vi "R4Master.vi"(6 "LabVIEW Web Service":refnum<class "Web Service.lvclass">=refnum) -> ()   [LabVIEW 2016]
uses:
  <vilib>/wsapi/Web Service.lvclass
  R4Controls/R4SBR_SetParams.ctl
  Controls/pH_SetParams Standard.ctl
  <vilib>/Platform/TimedLoop/XDataNode/timing_clust.ctl
  <vilib>/Platform/TimedLoop/XDataNode/nitl_modes.ctl
  <vilib>/Platform/TimedLoop/XDataNode/wakeup.ctl
  <vilib>/Platform/TimedLoop/XDataNode/loadnilvce.vi
  <vilib>/Platform/TimedLoop/XDataNode/XDataNode.xnode
  <vilib>/Platform/TimedLoop/XDataNode/XDNodeRunTimeDep.lvlib
panel:
  out "?":cluster{"Value":dbl, "Value":dbl}(graph)
  in  "R4SBR_Manual":T1
  out "error out":errorcluster
  out "error out (DATA COLLECT)":errorcluster
  out "error out (SBR)":errorcluster
  in  "R4SBR_SetParams":T2=[{"Phase"="Plug Feed", "Time, min"=0.0, "SBR_Manual (Standard)"={"Media Pump"=TRUE, "Water Pump"=TRUE, "Gas Pump"=FALSE, "Effluent Pump"=FALSE, "Release Pump"=FALSE}}, {"Phase"="Mixed Feed", "Time, min"=135.0, "SBR_Manual (Standard)"={"Media Pump"=TRUE, "Water Pump"=TRUE, "Gas Pump"=TRUE, "Effluent Pump"=FALSE, "Release Pump"=FALSE}}, {"Phase"="Mixed w/o Feed", "Time, min"=92.0, "SBR_Manual (Standard)"={"Media Pump"=FALSE, "Water Pump"=FALSE, "Gas Pump"=TRUE, "Effluent Pump"=FALSE, "Release Pump"=FALSE}}, {"Phase"="Settle", "Time, min"=7.0, "SBR_Manual (Standard)"={"Media Pump"=FALSE, "Water Pump"=FALSE, "Gas Pump"=FALSE, "Effluent Pump"=FALSE, "Release Pump"=TRUE}}, {"Phase"="Decant", "Time, min"=5.0, "SBR_Manual (Standard)"={"Media Pump"=FALSE, "Water Pump"=FALSE, "Gas Pump"=FALSE, "Effluent Pump"=TRUE, "Release Pump"=TRUE}}, {"Phase"="Idle", "Time, min"=1.0, "SBR_Manual (Standard)"={"Media Pump"=FALSE, "Water Pump"=FALSE, "Gas Pump"=FALSE, "Effluent Pump"=FALSE, "Release Pump"=FALSE}}]
  in  "R4 SBR_Switch":bool
  in  "R4DOSetParams":T3={"Set Point, mg/L"=0.0, "Tolerance, mg/L"=0.05, "N2 Valve Gain"=5000.0, "Air Valve Gain"=1000.0}
  in  "R4DOManual":cluster{"Air MFC":dbl, "N2 MFC":dbl} {"Air MFC" scale=0.0..500.0; "N2 MFC" scale=0.0..500.0}
  in  "R4 DO_Switch":bool=TRUE
  out "R4DO":cluster{"Signal":dbl, "Value":dbl}={"Signal"=0.012310571769960223, "Value"=5.584491888741017}
  in  "R4 pH_Switch":bool=TRUE
  in  "R4 pH_SetParams":T4={"Set Point"=7.5, "Tolerance"=0.1, "Pump Time On, secs"=6.0}
  in  "R4pH_Manual":cluster{"Acid Pump":bool, "Base Pump":bool}
  out "pH":cluster{"Signal":dbl, "Value":dbl}={"Signal"=0.0127343038254794, "Value"=7.4567616069444576}
  out "Timestamp":string="09/22/2017 10:45:23.660"
  out "Status":string="Off"
  out "Cycle Time Elapsed":dbl
  out "Phase Time Elapsed":dbl
  # "Use the web service input terminal to call the VIs on the Service subpalette of the Web Services palette. Do not remove it from the connector pane unless you don't need access to the palette."
  # "Any additional terminals added to the connector pane of a startup VI will be ignored."
  # "DO Control"
  # "SBR Control"
  # "If On, Automate SBR Cycle"
  # "pH Control"
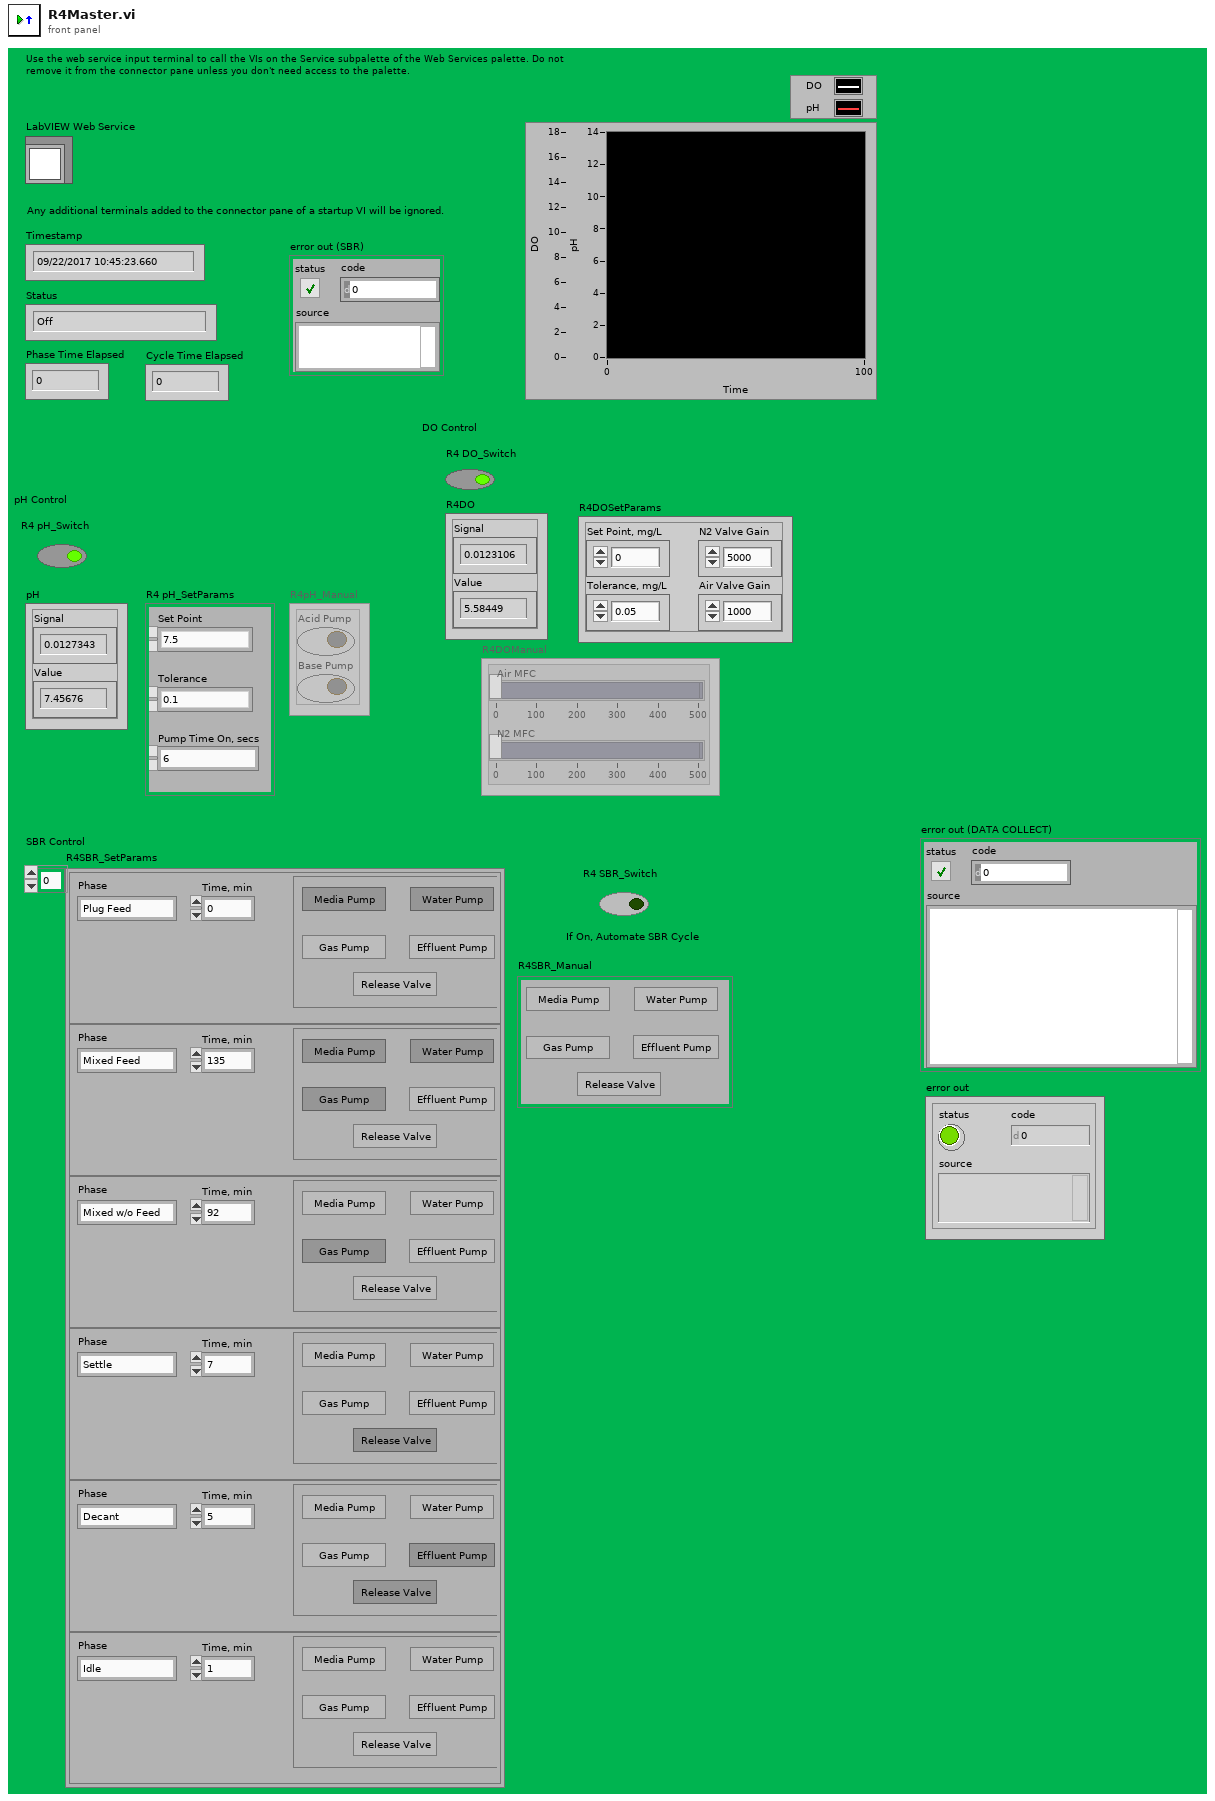
[diagram p1: front panel]
types:
  T1 = cluster{"Media Pump":bool, "Water Pump":bool, "Gas Pump":bool, "Effluent Pump":bool, "Release Pump":bool}
  T2 = typedef "R4SBR_SetParams.ctl" = cluster{"Phase":string, "Time, min":dbl, "SBR_Manual (Standard)":cluster{"Media Pump":bool, "Water Pump":bool, "Gas Pump":bool, "Effluent Pump":bool, "Release Pump":bool}}[]
  T3 = cluster{"Set Point, mg/L":dbl, "Tolerance, mg/L":dbl, "N2 Valve Gain":dbl, "Air Valve Gain":dbl}
  T4 = typedef "pH_SetParams Standard.ctl" = cluster{"Set Point":dbl, "Tolerance":dbl, "Pump Time On, secs":dbl}
  T5 = typedef "XDNodeRunTimeDep.lvlib/timing_clust.ctl" = cluster{"Expected End [f-1]":u64, "Actual End [f-1]":u64, "Finished Late? [f-1]":bool, "Expected End [i-1]":u64, "Actual End [i-1]":u64, "Finished Late? [i-1]":bool, "Expected Start [i]":u64, "Actual Start [i]":u64, "Expected Start [f]":u64, "Actual Start [f]":u64, "Source Name":string, "Structure Name":string, "Period":i64, "Deadline":i64, "Offset":i64, "Start":i64, "Priority":i32, "Timeout":i32, "Mode":T6, "Wakeup Reason":T7, "Error":errorcluster, "Source Type":string, "Secondary Source Type":string, "Global End Time":u64, "Global Start Time":u64, "Frame Duration":u64, "Iteration Duration":u64, "Assigned CPU":i32, "I/O Scan Engine Mode":u32}
  T6 = typedef "XDNodeRunTimeDep.lvlib/nitl_modes.ctl" = enum32{"No Change", "Process missed periods, maintain original phase", "Discard missed periods, maintain original phase", "Process missed periods, ignore original phase", "Discard missed periods, ignore original phase"}
  T7 = typedef "XDNodeRunTimeDep.lvlib/wakeup.ctl" = enum32{"Normal", "Aborted", "Asynchronous wakeup", "Timing source error", "Timed loop error", "Timeout"}
  T8 = cluster{"Media Pump":bool, "Water Pump":bool, "Effluent Pump":bool, "Release Valve":bool, "Gas Pump":bool}
  T9 = enum8{"Enabled", "Disabled", "Disabled and Grayed Out"}
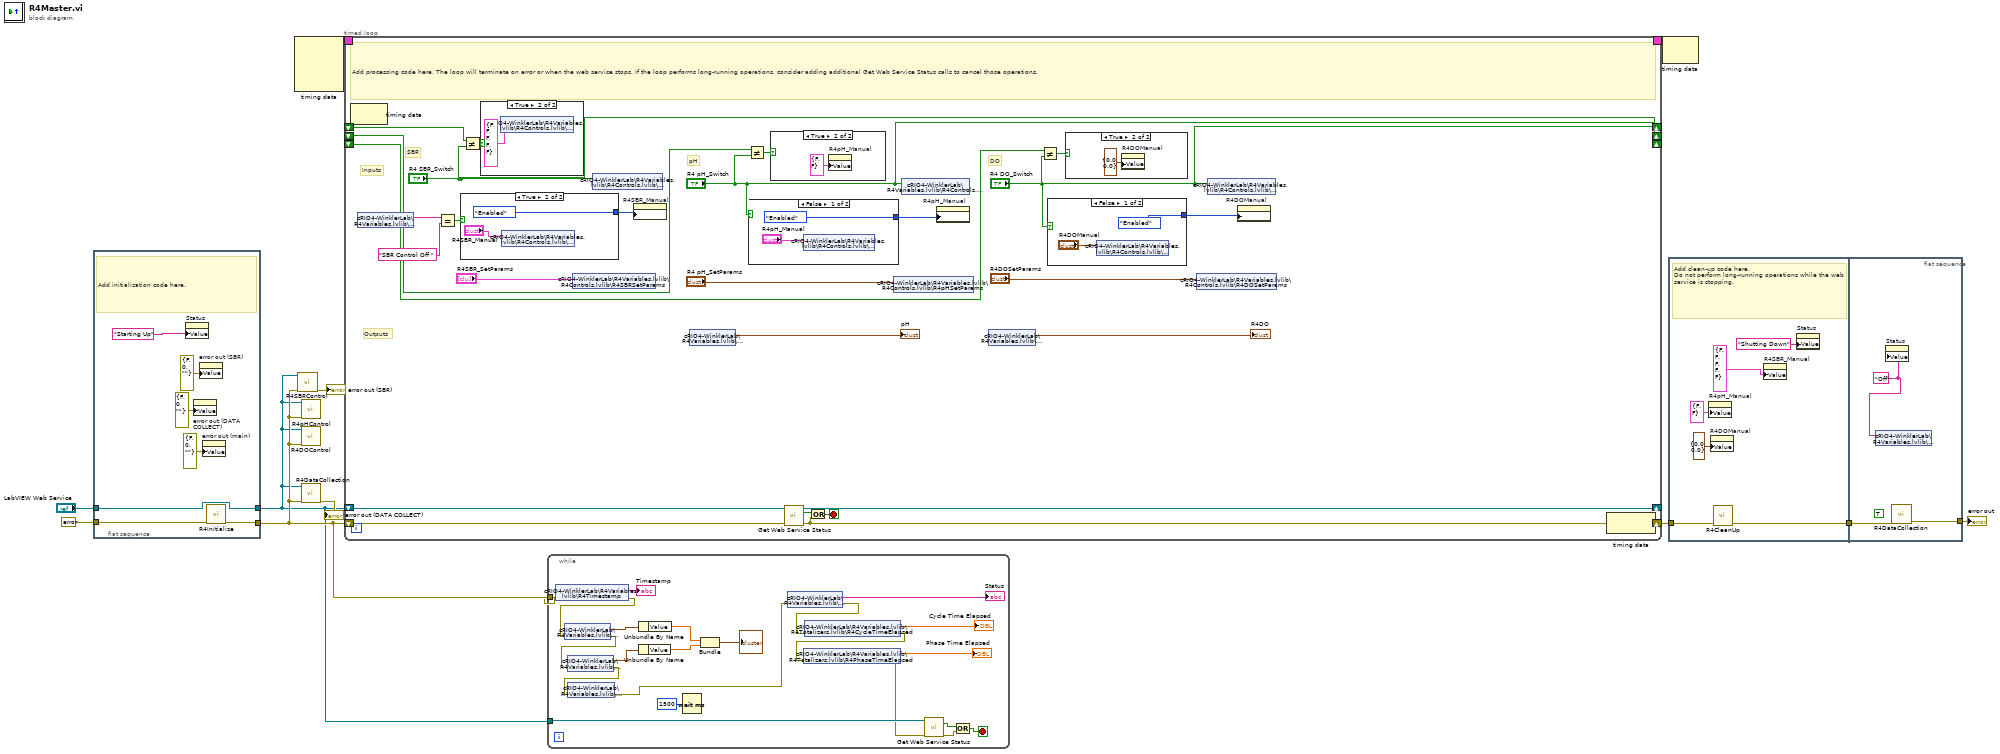
[diagram p0: block diagram]
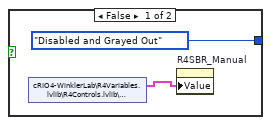
[diagram p5: hidden frame]
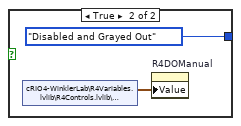
[diagram p6: hidden frame]
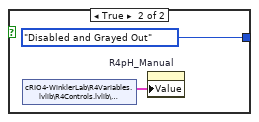
[diagram p7: hidden frame]
diagram:
  n1 = flat-sequence {
    tunnel: "LabVIEW Web Service" -> [w16]
    tunnel: errorcluster {"status"=FALSE, "code"=0, "source"=""} ("error constant") -> [w18]
    tunnel: [w17] -> w3
    tunnel: [w16] -> w1
    frame #0 {
      # "Add initialization code here."
      n2 = property on="Status" class="Str"("Value"="Starting Up" ("Status")) -> ()  [unwired: 2 in, 2 out]
      n3 = property on="error out (DATA COLLECT)" class="Clust (strict)"("Value"=errorcluster {"status"=FALSE, "code"=0, "source"=""} ("error out (DATA COLLECT)")) -> ()  [unwired: 2 in, 2 out]
      n4 = property on="error out (SBR)" class="Clust (strict)"("Value"=errorcluster {"status"=FALSE, "code"=0, "source"=""} ("error out (SBR)")) -> ()  [unwired: 2 in, 2 out]
      n5 = property on="error out (main)" class="Clust (strict)"("Value"=errorcluster {"status"=FALSE, "code"=0, "source"=""} ("error out")) -> ()  [unwired: 2 in, 2 out]
      n6 = call "R4Initialize.vi"("error in (no error)"=w18) -> ("error out"=w17:errorcluster)  [unwired: 10 in]
    }
  }
  n7 = node-c288() -> (w8:T5)  [unwired: 4 in]
  n8 = call "R4SBRControl.vi"("error constant"=w3, "LabVIEW Web Service"=w1) -> ("error out"=→"error out (SBR)":errorcluster)  [unwired: 9 in]
  n9 = call "R4pHControl.vi"("error constant"=w3, "LabVIEW Web Service"=w1) -> ()  [unwired: 10 in]
  n10 = call "R4DOControl.vi"("error constant"=w3, "LabVIEW Web Service"=w1) -> ()  [unwired: 10 in]
  n11 = call "R4DataCollection.vi"("error constant"=w3, "LabVIEW Web Service"=w1) -> ("error out"=→"error out (DATA COLLECT)":errorcluster)  [unwired: 9 in]
  n12 = timed-loop {
    shift-right: [w42] -> w9
    shift-left: w3 -> [w41]
    shift-right: [w39] -> _
    shift-left: w1 -> [w39]
    timing: w8 -> [_]
    timing-out: [_] -> w7
    shift-right: ["R4 SBR_Switch"] -> _
    shift-left: _ -> [w29]
    shift-right: ["R4 pH_Switch"] -> _
    shift-left: _ -> [w35]
    shift-right: ["R4 DO_Switch"] -> _
    shift-left: _ -> [w33]
    stop <- w40 stop-if-true
    # "DO"
    # "pH"
    # "Outputs"
    # "Inputs"
    # "SBR"
    # "Add processing code here. The loop will terminate on error or when the web service stops. If the loop performs long-running operations, consider adding additional Get Web Service Status calls to cancel those operations."
    n13 = node-c288() -> ()  [unwired: 1 in, 1 out]
    n14 = shared-variable "cRIO4-WinklerLab\\R4Variables.lvlib\\R4Status"() -> (w28:string)  [unwired: 1 in, 1 out]
    n15 = Equal?(x=w28, y="SBR Control Off " ("string")) -> (x = y?=w30:bool)
    n16 = case shown="True" w30 {
      tunnel: [T9."Disabled and Grayed Out" ("Disabled") T9."Enabled" ("Disabled")] -> w19
      frame False {
        n17 = shared-variable "cRIO4-WinklerLab\\R4Variables.lvlib\\R4Controls.lvlib\\R4SBRManual"() -> (w47:T1)  [unwired: 1 in, 1 out]
        n18 = property on="R4SBR_Manual" class="Clust (strict)"("Value"=w47) -> ()  [unwired: 2 in, 2 out]
      }
      frame True {
        n19 = shared-variable "cRIO4-WinklerLab\\R4Variables.lvlib\\R4Controls.lvlib\\R4SBRManual"("R4SBR_Manual") -> ()  [unwired: 1 in, 1 out]
      }
    }
    n20 = Not Equal?(x=w29, y="R4 SBR_Switch") -> (x != y?=w36:bool)
    n21 = case shown="True" w36 {
      frame False {
      }
      frame True {
        n22 = shared-variable "cRIO4-WinklerLab\\R4Variables.lvlib\\R4Controls.lvlib\\R4SBRManual"(T8 {"Media Pump"=FALSE, "Water Pump"=FALSE, "Effluent Pump"=FALSE, "Release Valve"=FALSE, "Gas Pump"=FALSE} ("R4SBRManual")) -> ()  [unwired: 1 in, 1 out]
      }
    }
    n23 = shared-variable "cRIO4-WinklerLab\\R4Variables.lvlib\\R4Controls.lvlib\\R4SBRSetParams"("R4SBR_SetParams") -> ()  [unwired: 1 in, 1 out]
    n24 = shared-variable "cRIO4-WinklerLab\\R4Variables.lvlib\\R4Controls.lvlib\\R4SBRSwitch"("R4 SBR_Switch") -> ()  [unwired: 1 in, 1 out]
    n25 = property on="R4SBR_Manual" class="Clust (strict)"("DisabledEnum"=w19) -> ()  [unwired: 2 in, 2 out]
    n26 = shared-variable "cRIO4-WinklerLab\\R4Variables.lvlib\\R4Signals.lvlib\\R4pH"() -> (→"pH":cluster{"Signal":dbl, "Value":dbl})  [unwired: 1 in, 1 out]
    n27 = Not Equal?(x=w35, y="R4 pH_Switch") -> (x != y?=w34:bool)
    n28 = case shown="False" "R4 pH_Switch" {
      tunnel: [T9."Enabled" ("Disabled") T9."Disabled and Grayed Out" ("Disabled")] -> w38
      frame False {
        n29 = shared-variable "cRIO4-WinklerLab\\R4Variables.lvlib\\R4Controls.lvlib\\R4pHManual"("R4pH_Manual") -> ()  [unwired: 1 in, 1 out]
      }
      frame True {
        n30 = shared-variable "cRIO4-WinklerLab\\R4Variables.lvlib\\R4Controls.lvlib\\R4pHManual"() -> (w57:cluster{"Acid Pump":bool, "Base Pump":bool})  [unwired: 1 in, 1 out]
        n31 = property on="R4pH_Manual" class="Clust (strict)"("Value"=w57) -> ()  [unwired: 2 in, 2 out]
      }
    }
    n32 = case shown="True" w34 {
      frame False {
      }
      frame True {
        n33 = property on="R4pH_Manual" class="Clust (strict)"("Value"=cluster{"Acid Pump":bool, "Base Pump":bool} {"Acid Pump"=FALSE, "Base Pump"=FALSE} ("R1pH_Manual")) -> ()  [unwired: 2 in, 2 out]
      }
    }
    n34 = call <vilib>:"Get Web Service Status.vi"("LabVIEW Web Service"=w39, "error in (no error)"=w41) -> ("service stopping?"=w43:bool, "error out"=w42:errorcluster)  [unwired: 11 in, 1 out]
    n35 = Or(x=w43, y=w42) -> (x .or. y?=w40:bool)
    n36 = shared-variable "cRIO4-WinklerLab\\R4Variables.lvlib\\R4Controls.lvlib\\R4pHSetParams"("R4 pH_SetParams") -> ()  [unwired: 1 in, 1 out]
    n37 = shared-variable "cRIO4-WinklerLab\\R4Variables.lvlib\\R4Controls.lvlib\\R4pHSwitch"("R4 pH_Switch") -> ()  [unwired: 1 in, 1 out]
    n38 = property on="R4pH_Manual" class="Clust (strict)"("DisabledEnum"=w38) -> ()  [unwired: 2 in, 2 out]
    n39 = shared-variable "cRIO4-WinklerLab\\R4Variables.lvlib\\R4Signals.lvlib\\R4DO"() -> (→"R4DO":cluster{"Signal":dbl, "Value":dbl})  [unwired: 1 in, 1 out]
    n40 = Not Equal?(x=w33, y="R4 DO_Switch") -> (x != y?=w32:bool)
    n41 = case shown="False" "R4 DO_Switch" {
      tunnel: [T9."Enabled" ("Disabled") T9."Disabled and Grayed Out" ("Disabled")] -> w37
      frame False {
        n42 = shared-variable "cRIO4-WinklerLab\\R4Variables.lvlib\\R4Controls.lvlib\\R4DOManual"("R4DOManual") -> ()  [unwired: 1 in, 1 out]
      }
      frame True {
        n43 = shared-variable "cRIO4-WinklerLab\\R4Variables.lvlib\\R4Controls.lvlib\\R4DOManual"() -> (w53:cluster{"Air MFC":dbl, "N2 MFC":dbl})  [unwired: 1 in, 1 out]
        n44 = property on="R4DOManual" class="Clust (strict)"("Value"=w53) -> ()  [unwired: 2 in, 2 out]
      }
    }
    n45 = case shown="True" w32 {
      frame False {
      }
      frame True {
        n46 = property on="R4DOManual" class="Clust (strict)"("Value"=cluster{"Air MFC":dbl, "N2 MFC":dbl} {"Air MFC"=0.0, "N2 MFC"=0.0} ("R1DOManual")) -> ()  [unwired: 2 in, 2 out]
      }
    }
    n47 = shared-variable "cRIO4-WinklerLab\\R4Variables.lvlib\\R4Controls.lvlib\\R4DOSetParams"("R4DOSetParams") -> ()  [unwired: 1 in, 1 out]
    n48 = shared-variable "cRIO4-WinklerLab\\R4Variables.lvlib\\R4Controls.lvlib\\R4DOSwitch"("R4 DO_Switch") -> ()  [unwired: 1 in, 1 out]
    n49 = property on="R4DOManual" class="Clust (strict)"("DisabledEnum"=w37) -> ()  [unwired: 2 in, 2 out]
    n50 = node-c288() -> ()  [unwired: 1 in, 1 out]
  }
  n51 = while {
    tunnel: w1 -> [w81]
    tunnel: w3 -> [w75]
    stop <- w78 stop-if-true
    n52 = shared-variable "cRIO4-WinklerLab\\R4Variables.lvlib\\R4Timestamp"(error in=w75) -> (→"Timestamp":string, error out=w73:errorcluster)
    n53 = shared-variable "cRIO4-WinklerLab\\R4Variables.lvlib\\R4Signals.lvlib\\R4DO"(error in=w73) -> (w72:cluster{"Signal":dbl, "Value":dbl}, error out=w71:errorcluster)
    n54 = shared-variable "cRIO4-WinklerLab\\R4Variables.lvlib\\R4Signals.lvlib\\R4pH"(error in=w71) -> (w70:cluster{"Signal":dbl, "Value":dbl}, error out=w62:errorcluster)
    n55 = shared-variable "cRIO4-WinklerLab\\R4Variables.lvlib\\R4Signals.lvlib\\R4Off"(error in=w62) -> (error out=w61:errorcluster)  [unwired: 1 out]
    n56 = Unbundle By Name(w70) -> ("Value"=w74:dbl)
    n57 = Unbundle By Name(w72) -> ("Value"=w82:dbl)
    n58 = Wait (ms)(milliseconds to wait=u32 1500) -> ()  [unwired: 1 out]
    n59 = Bundle("Value"=w82, "Value"=w74) -> (→"?":cluster{"Value":dbl, "Value":dbl})  [unwired: 1 in]
    n60 = shared-variable "cRIO4-WinklerLab\\R4Variables.lvlib\\R4Status"(error in=w61) -> (→"Status":string, error out=w68:errorcluster)
    n61 = shared-variable "cRIO4-WinklerLab\\R4Variables.lvlib\\R4Totalizers.lvlib\\R4CycleTimeElapsed"(error in=w68) -> (→"Cycle Time Elapsed":dbl, error out=w66:errorcluster)
    n62 = shared-variable "cRIO4-WinklerLab\\R4Variables.lvlib\\R4Totalizers.lvlib\\R4PhaseTimeElapsed"(error in=w66) -> (→"Phase Time Elapsed":dbl, error out=w65:errorcluster)
    n63 = call <vilib>:"Get Web Service Status.vi"("LabVIEW Web Service"=w81, "error in (no error)"=w65) -> ("service stopping?"=w80:bool, "error out"=w79:errorcluster)  [unwired: 11 in, 1 out]
    n64 = Or(x=w80, y=w79) -> (x .or. y?=w78:bool)
  }
  n65 = node-c288(w7) -> ()  [unwired: 1 out]
  n66 = flat-sequence {
    tunnel: w9 -> [w84]
    tunnel: [w83] -> w5
    tunnel: w5 -> [w91]
    tunnel: [w90] -> w4
    frame #0 {
      # "Add clean-up code here.\nDo not perform long-running operations while the web service is stopping."
      n67 = property on="R4pH_Manual" class="Clust (strict)"("Value"=cluster{"Acid Pump":bool, "Base Pump":bool} {"Acid Pump"=FALSE, "Base Pump"=FALSE} ("R1pH_Manual")) -> ()  [unwired: 2 in, 2 out]
      n68 = property on="R4DOManual" class="Clust (strict)"("Value"=cluster{"Air MFC":dbl, "N2 MFC":dbl} {"Air MFC"=0.0, "N2 MFC"=0.0} ("R1DOManual")) -> ()  [unwired: 2 in, 2 out]
      n69 = call "R4CleanUp.vi"("error in (no error)"=w84) -> ("error out"=w83:errorcluster)  [unwired: 10 in]
      n70 = property on="R4SBR_Manual" class="Clust (strict)"("Value"=T8 {"Media Pump"=FALSE, "Water Pump"=FALSE, "Effluent Pump"=FALSE, "Release Valve"=FALSE, "Gas Pump"=FALSE} ("R4SBRManual")) -> ()  [unwired: 2 in, 2 out]
      n71 = property on="Status" class="Str"("Value"="Shutting Down" ("Status")) -> ()  [unwired: 2 in, 2 out]
    }
    frame #1 {
      w89 = "Off" ("Status")
      (unwired) TRUE ("Write Once")
      n72 = shared-variable "cRIO4-WinklerLab\\R4Variables.lvlib\\R4Status"(w89) -> ()  [unwired: 1 in, 1 out]
      n73 = property on="Status" class="Str"("Value"=w89) -> ()  [unwired: 2 in, 2 out]
      n74 = call "R4DataCollection.vi"("error constant"=w91) -> ("error out"=w90:errorcluster)  [unwired: 10 in]
    }
  }
  "error out" <- w4
